vi "Inline - Update Status Channels - Get Index and Value from Channel Name.vi"(9 "Time (us)/Error Counter Value":u32, 10 "Error Code":i32, 11 "Status Channel":T1) -> (2 "Value":dbl, 3 "index":i32)   [LabVIEW 2019, in "Ballard MIL-1553 Engine.lvlib"]
uses:
  Ballard MIL-1553 Engine.lvlib
  Controls/Inline_Status_Channels.ctl
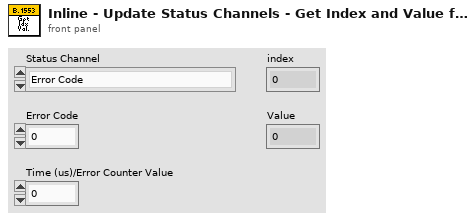
[diagram p1: front panel]
types:
  T1 = typedef "Ballard MIL-1553 Engine.lvlib/Inline_Status_Channels.ctl" = enum16{"Error Code", "Inline Read Time (us)", "Inline Write Time (us)", "Unconfigured Frames Counter", "Monitor - Error Counter", "General Protocol Error Counter", "Wrong Sync Error Counter", "Improper Number of Data Words Error", "Manchester Error Counter", "Parity Error Counter", "Word Error Counter"}
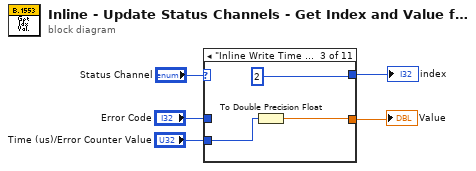
[diagram p0: block diagram]
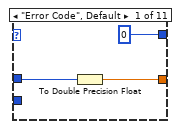
[diagram p2: hidden frame]
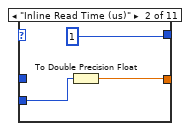
[diagram p3: hidden frame]
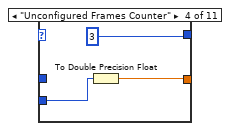
[diagram p4: hidden frame]
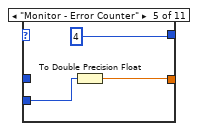
[diagram p5: hidden frame]
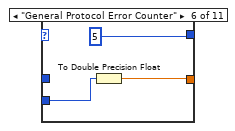
[diagram p6: hidden frame]
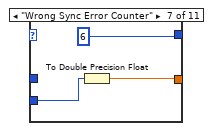
[diagram p7: hidden frame]
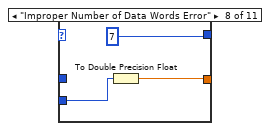
[diagram p8: hidden frame]
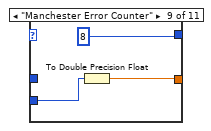
[diagram p9: hidden frame]
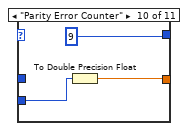
[diagram p10: hidden frame]
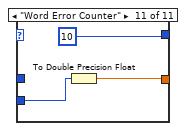
[diagram p11: hidden frame]
diagram:
  n1 = case shown="\"Inline Write Time (us)\"" "Status Channel" {
    tunnel: [0 ("index") 1 ("index") 2 ("index") 3 ("index") 4 ("index") 5 ("index") 6 ("index") 7 ("index") 8 ("index") 9 ("index") 10 ("index")] -> w1
    tunnel: "Error Code" -> [w7 _ _ _ _ _ _ _ _ _ _]
    tunnel: [w6 w10 w13 w16 w19 w22 w25 w28 w31 w34 w37] -> w4
    tunnel: "Time (us)/Error Counter Value" -> [_ w9 w12 w15 w18 w21 w24 w27 w30 w33 w36]
    frame "Error Code", Default {
      n2 = To Double Precision Float(number=w7) -> (double precision float=w6:dbl)
    }
    frame "Inline Read Time (us)" {
      n3 = To Double Precision Float(number=w9) -> (double precision float=w10:dbl)
    }
    frame "Inline Write Time (us)" {
      n4 = To Double Precision Float(number=w12) -> (double precision float=w13:dbl)
    }
    frame "Unconfigured Frames Counter" {
      n5 = To Double Precision Float(number=w15) -> (double precision float=w16:dbl)
    }
    frame "Monitor - Error Counter" {
      n6 = To Double Precision Float(number=w18) -> (double precision float=w19:dbl)
    }
    frame "General Protocol Error Counter" {
      n7 = To Double Precision Float(number=w21) -> (double precision float=w22:dbl)
    }
    frame "Wrong Sync Error Counter" {
      n8 = To Double Precision Float(number=w24) -> (double precision float=w25:dbl)
    }
    frame "Improper Number of Data Words Error" {
      n9 = To Double Precision Float(number=w27) -> (double precision float=w28:dbl)
    }
    frame "Manchester Error Counter" {
      n10 = To Double Precision Float(number=w30) -> (double precision float=w31:dbl)
    }
    frame "Parity Error Counter" {
      n11 = To Double Precision Float(number=w33) -> (double precision float=w34:dbl)
    }
    frame "Word Error Counter" {
      n12 = To Double Precision Float(number=w36) -> (double precision float=w37:dbl)
    }
  }
  "Value" <- w4
  "index" <- w1
